vi "Direct Message Sent.vi"(8 "error in (no error)":errorcluster, 10 "Message":T1, 11 "Chat Window Model in":refnum<class "Chat Window Model.lvclass">) -> (0 "error out":errorcluster, 3 "Chat Window Model out":refnum<class "Chat Window Model.lvclass">)   [LabVIEW 2020, in "Chat Window Model.lvlib" / "Chat Window Model.lvclass"]
uses:
  Chat Window Model.lvclass
  C:/Program Files/National Instruments/LabVIEW 2020/vi.lib/ActorFramework/Actor/Actor.lvclass
  Controls/Message Control.ctl
  <vilib>/ActorFramework/Actor/Actor.lvclass/Actor.ctl
  <vilib>/ActorFramework/Message Enqueuer/Message Enqueuer.lvclass/Message Enqueuer.ctl
  Chat Window Model.lvclass/Chat Window Model.ctl
  Chat Window Model Messages/Preserve Sent Message Msg/Preserve Sent Message Msg.lvclass/Preserve Sent Message Msg.ctl
  Msg Forward Interface Actor/Msg Forward Interface Actor Messages/Direct Message Sent Msg/Direct Message Sent Msg.lvclass/Direct Message Sent Msg.ctl
  <vilib>/ActorFramework/Message Enqueuer/Init from Existing Queue.vi
  <vilib>/ActorFramework/Message Enqueuer/Enqueue.vi
  Chat Window Model Messages/Preserve Sent Message Msg/Preserve Sent Message Msg.lvclass
  C:/Program Files/National Instruments/LabVIEW 2020/vi.lib/ActorFramework/Message/Message.lvclass
  Msg Forward Interface Actor/Msg Forward Interface Actor Messages/Direct Message Sent Msg/Direct Message Sent Msg.lvclass
  <vilib>/ActorFramework/Message Priority Queue/Priority Enqueue.vi
  <vilib>/ActorFramework/Message Enqueuer/Message Enqueuer.lvclass
  <vilib>/ActorFramework/Actor/Actor.lvclass
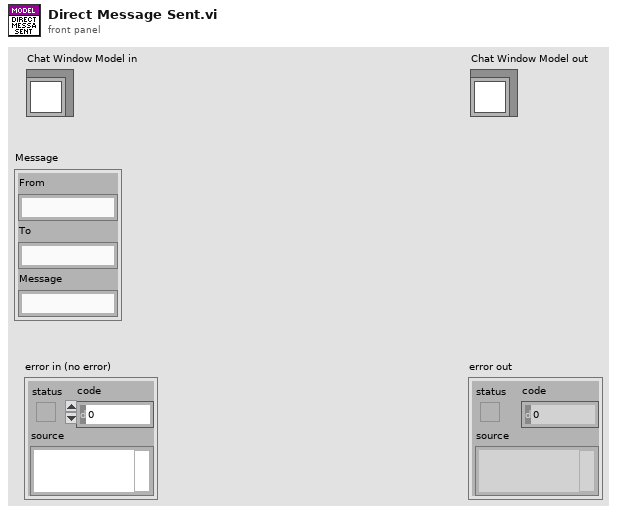
[diagram p1: front panel]
types:
  T1 = typedef "Message Control.ctl" = cluster{"From":string, "To":string, "Message":string}
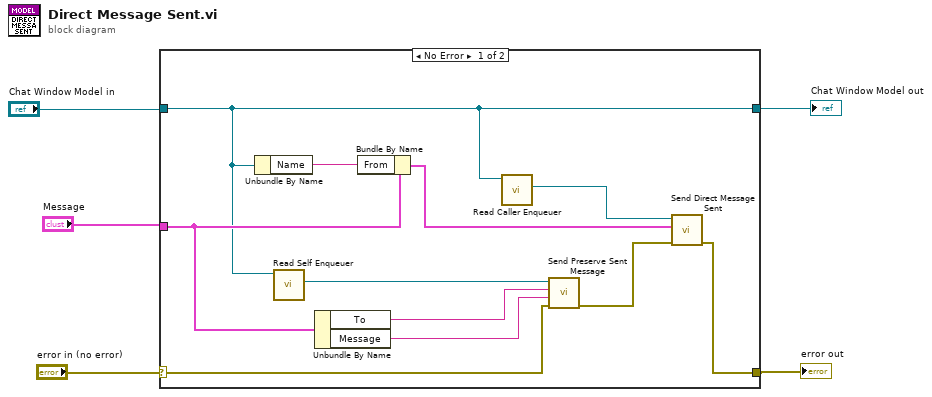
[diagram p0: block diagram]
diagram:
  n1 = case shown="No Error" "error in (no error)" {
    selector: "error in (no error)" -> [w12 w18]
    tunnel: [w8 w18] -> w4
    tunnel: [w11 w17] -> w1
    tunnel: "Chat Window Model in" -> [w11 w17]
    tunnel: "Message" -> [w15 _]
    frame No Error {
      n2 = Unbundle By Name(w11) -> ("Name"=w16:string)
      n3 = call <vilib>:"Read Self Enqueuer.vi"("Actor"=w11) -> ("Self Enqueuer"=w10:refnum<class "Message Enqueuer.lvclass">)  [unwired: 10 in]
      n4 = Unbundle By Name(w15) -> ("To"=w13:string, "Message"=w14:string)
      n5 = Bundle By Name(cluster=w15, "From"=w16) -> (w6:T1)
      n6 = call <vilib>:"Read Caller Enqueuer.vi"("Actor"=w11) -> ("Caller Enqueuer"=w9:refnum<class "Message Enqueuer.lvclass">)  [unwired: 10 in]
      n7 = call "Send Preserve Sent Message.vi"("error in (no error)"=w12, "Sent Message"=w14, "To"=w13, "Message Enqueuer"=w10) -> ("error out"=w7:errorcluster)  [unwired: 6 in, 1 out]
      n8 = call "Send Direct Message Sent.vi"("error in (no error)"=w7, "Message"=w6, "Message Enqueuer"=w9) -> ("error out"=w8:errorcluster)  [unwired: 7 in, 1 out]
    }
    frame Error {
    }
  }
  "error out" <- w4
  "Chat Window Model out" <- w1
